vi "TEG P116x2_Write_Manual.vi"(8 "error in (no error)":errorcluster, 9 "RateSP":T2, 10 "NuevoSP":T2, 11 "Comunicaciones":T1={"Alicats"="ASRL6::INSTR", "Alic"=FALSE, "eValve"="ASRL6::INSTR", "eval"=FALSE, "Eurotherm"="ASRL6::INSTR", "euro"=FALSE, "Cell GAS"="ASRL6::INSTR", "cgas"=FALSE, "Cell H2S"="ASRL6::INSTR", "ch2s"=FALSE}) -> (0 "error out":errorcluster, 1 "RateSP(C/min) 2":T2, 2 "NuevoSP(C) 2":T2)   [LabVIEW 2017]
uses:
  2xP116.ctl
  REACTOR_COMUNICACIONES.ctl
  Eurotherm_New_Module.ctl
  REACTOR_GLOBALES.vi
panel:
  out "PV":T2
  out "WorkingSP":T2
  out "TargetSP":T2
  in  "Cancel":bool
  in  "Write":bool
  out "Enable(T)":bool=TRUE
  out "VISA Promux":refnum<visa-resource-name>
  in  "Delay Time (s)":dbl=0.1
  # "Programando controladores P116"
  # "C"
  # "CALOR"
  # "C/min"
  # "C"
  # "FRIO"
  # "C/min"
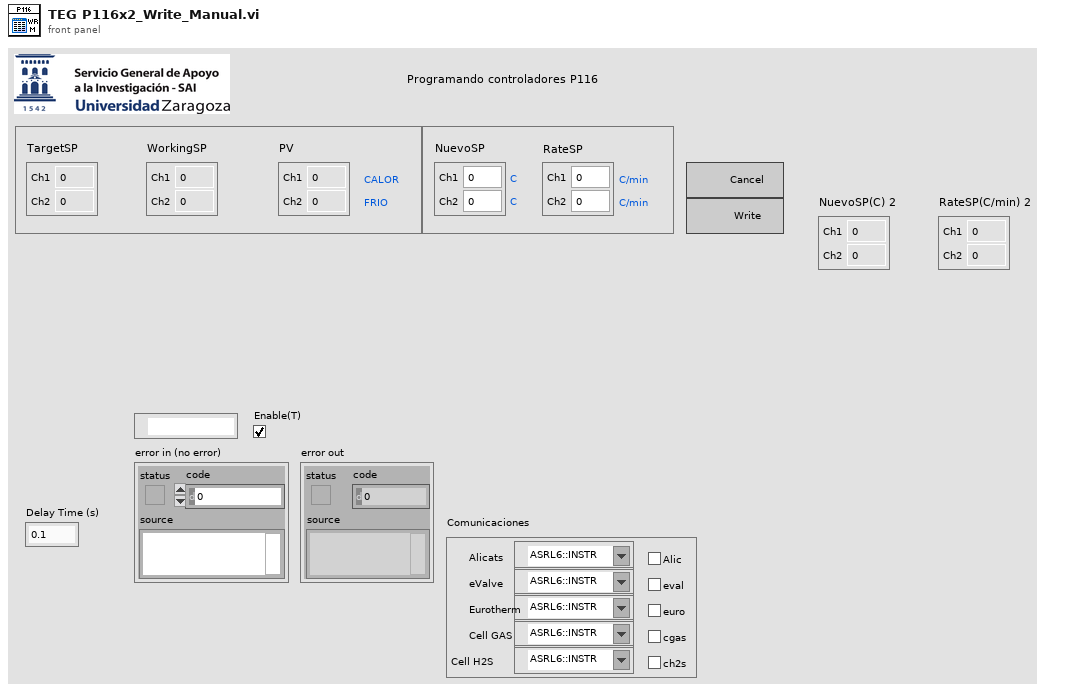
[diagram p1: front panel]
types:
  T1 = typedef "REACTOR_COMUNICACIONES.ctl" = cluster{"Alicats":refnum<visa-resource-name>, "Alic":bool, "eValve":refnum<visa-resource-name>, "eval":bool, "Eurotherm":refnum<visa-resource-name>, "euro":bool, "Cell GAS":refnum<visa-resource-name>, "cgas":bool, "Cell H2S":refnum<visa-resource-name>, "ch2s":bool}
  T2 = typedef "2xP116.ctl" = cluster{"Ch1":dbl, "Ch2":dbl}
  T3 = typedef "TEG P116x2.ctl" = cluster{"TargetSP":T2, "WorkingSP":T2, "Temperatura":T2, "Error":bool, "Date":string, "Delay(s)":dbl, "RateSP":T2, "Potencia":T2}
  T4 = typedef "Eurotherm_New_Module.ctl" = enum16{"Initialize", "Write SP", "Read SP+PV", "Write Rate", "Set P", "Set I", "Set D", "Shutdown"}
  T5 = enum16{"Add 1", "Add 2", "Add 10", "Add 11", "Add 12", "Add 13"}[]
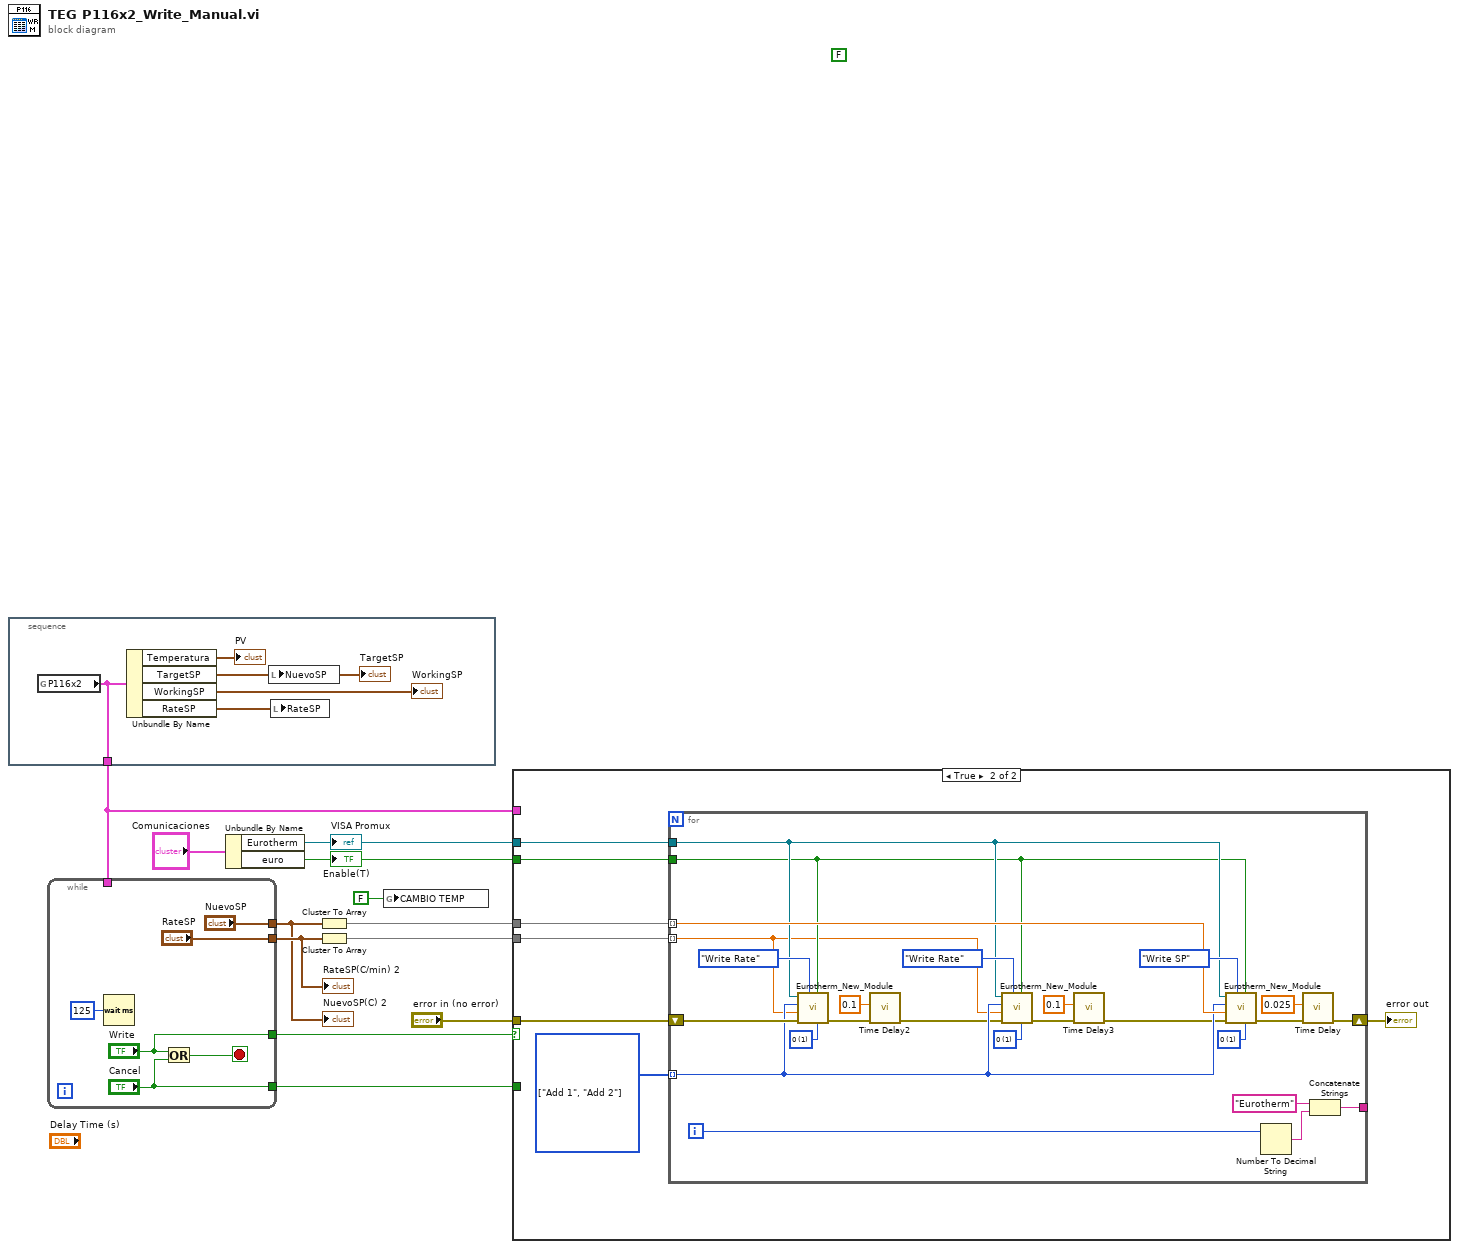
[diagram p0: block diagram]
diagram:
  (unwired) FALSE
  n1 = stacked-sequence {
    tunnel: [w14] -> w4
    frame #0 {
      n2 = global read "REACTOR_GLOBALES.vi" "P116x2"() -> (w14:T3)
      n3 = Unbundle By Name(w14) -> ("Temperatura"=→"PV":T2, "TargetSP"=w15:T2, "WorkingSP"=→"WorkingSP":T2, "RateSP"=w13:T2)
      "TargetSP" <- w15
      n4 = local write "NuevoSP"(w15) -> ()
      n5 = local write "RateSP"(w13) -> ()
    }
  }
  n6 = while {
    tunnel: ["Cancel"] -> w11
    tunnel: ["NuevoSP"] -> w2
    tunnel: ["RateSP"] -> w3
    tunnel: ["Write"] -> w7
    tunnel: w4 -> [_]
    stop <- w18 stop-if-true
    n7 = Wait (ms)(milliseconds to wait=u32 125) -> ()  [unwired: 1 out]
    n8 = Or(x="Write", y="Cancel") -> (x .or. y?=w18:bool)
  }
  "NuevoSP(C) 2" <- w2
  "RateSP(C/min) 2" <- w3
  n9 = Unbundle By Name("Comunicaciones") -> ("Eurotherm"=w5:refnum<visa-resource-name>, "euro"=w12:bool)
  "Enable(T)" <- w12
  "VISA Promux" <- w5
  n10 = Cluster To Array(cluster=w2) -> (array=w9:dbl[])
  n11 = Cluster To Array(cluster=w3) -> (array=w8:dbl[])
  n12 = global write "REACTOR_GLOBALES.vi" "CAMBIO TEMP"(FALSE ("ChangeT")) -> ()
  n13 = case shown="True" w7 {
    tunnel: w12 -> [_ w29]
    tunnel: w11 -> [_ _]
    tunnel: "error in (no error)" -> [_ w27]
    tunnel: w9 -> [_ w25]
    tunnel: w8 -> [_ w26]
    tunnel: w5 -> [_ w30]
    tunnel: w4 -> [_ _]
    frame False {
    }
    frame True {
      w24 = T5 [enum."Add 1", enum."Add 2"] items=["Add 1", "Add 2", "Add 10", "Add 11", "Add 12", "Add 13"]
      n14 = for {
        tunnel: w24 -> [w36] mode=indexing
        shift-right: [w46] -> w28
        shift-left: w27 -> [w50]
        tunnel: [w53] -> _
        tunnel: w25 -> [w48] mode=indexing
        tunnel: w26 -> [w31] mode=indexing
        tunnel: w30 -> [w33]
        tunnel: w29 -> [w32]
        i -> [w45]
        w38 = u16 1 items=["0"=1, "1"=10, "2"=100] ("Decimales")
        w44 = u16 1 items=["0"=1, "1"=10, "2"=100] ("Decimales")
        w43 = u16 1 items=["0"=1, "1"=10, "2"=100] ("Decimales")
        n15 = call "Eurotherm_New_Module.vi"("Decimales"=w44, "Eurotherm (T:Enable)"=w32, "Command"=Eurotherm_New_Module."Write Rate", "error in (no error)"=w50, "Value"=w31, "Address"=w36, "VISA resource name"=w33) -> ("error out"=w42:errorcluster)  [unwired: 3 in, 1 out]
        n16 = call "Time Delay2"("error in (no error)"=w42, "Delay Time (s)"=0.1) -> ("error out"=w35:errorcluster)  [unwired: 9 in]
        n17 = call "Eurotherm_New_Module.vi"("Decimales"=w38, "Eurotherm (T:Enable)"=w32, "Command"=Eurotherm_New_Module."Write Rate", "error in (no error)"=w35, "Value"=w31, "Address"=w36, "VISA resource name"=w33) -> ("error out"=w39:errorcluster)  [unwired: 3 in, 1 out]
        n18 = call "Time Delay3"("error in (no error)"=w39, "Delay Time (s)"=0.1) -> ("error out"=w34:errorcluster)  [unwired: 9 in]
        n19 = call "Eurotherm_New_Module.vi"("Decimales"=w43, "Eurotherm (T:Enable)"=w32, "Command"=Eurotherm_New_Module."Write SP", "error in (no error)"=w34, "Value"=w48, "Address"=w36, "VISA resource name"=w33) -> ("error out"=w47:errorcluster)  [unwired: 3 in, 1 out]
        n20 = Number To Decimal String(number=w45) -> (decimal integer string=w54:string)  [unwired: 1 in]
        n21 = call "Time Delay"("error in (no error)"=w47, "Delay Time (s)"=0.025) -> ("error out"=w46:errorcluster)  [unwired: 9 in]
        n22 = Concatenate Strings("Eurotherm" ("error source (\" \")"), w54) -> (w53:string)
      }
      "error out" <- w28
    }
  }
